vi "Lab01_LabViewSinusoidalWave_Bennett.vi"() -> ()   [LabVIEW 2017]
uses:
  <vilib>/Analysis/baseanly.llb/Mean (DBL).vi
  <vilib>/Analysis/5stat.llb/RMS (DBL).vi
  <vilib>/Analysis/NI_AALBase.lvlib
  <vilib>/Analysis/NI_AALPro.lvlib
panel:
  out "RMS":string
  out "Mean":string
  out "Min":string
  out "Max":string
  in  "Offset":dbl=1.0
  in  "Amplitude":dbl=1.0
  in  "Fraction of Radians":dbl
  in  "milliseconds to wait":u32
  in  "stop":bool
  out "Waveform Graph":dbl[](graph)
  # "09/06/17"
  # "ELEC3800: IoT                               Lab01                                                        Matt Bennett"
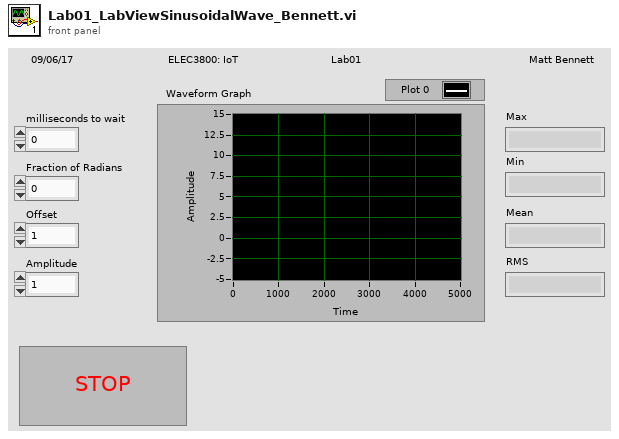
[diagram p1: front panel]
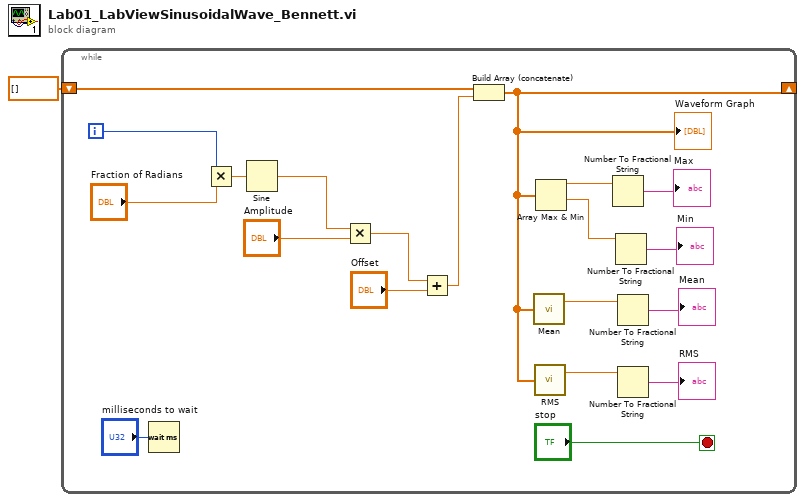
[diagram p0: block diagram]
diagram:
  n1 = while {
    shift-right: [w10] -> _
    shift-left: dbl[] [] -> [w21]
    i -> [w17]
    stop <- "stop" stop-if-true
    n2 = Wait (ms)(milliseconds to wait="milliseconds to wait") -> ()  [unwired: 1 out]
    n3 = Multiply(x=w17, y="Fraction of Radians") -> (x*y=w16:dbl)
    n4 = Sine(x=w16) -> (sin(x)=w14:dbl)
    n5 = Multiply(x=w14, y="Amplitude") -> (x*y=w12:dbl)
    n6 = Add(x=w12, y="Offset") -> (x+y=w11:dbl)
    n7 = Build Array (concatenate)(w21, w11) -> (w10:dbl[])
    "Waveform Graph" <- w10
    n8 = call-poly <vilib>:"Mean.vi"("X"=w10) -> ("mean"=w3:dbl)  [unwired: 1 out]
    n9 = call-poly <vilib>:"RMS.vi"("X"=w10) -> ("rms value"=w2:dbl)  [unwired: 1 out]
    n10 = Array Max & Min(array=w10) -> (max value=w9:dbl, min value=w4:dbl)  [unwired: 2 out]
    n11 = Number To Fractional String(number=w9) -> (F-format string=→"Max":string)  [unwired: 3 in]
    n12 = Number To Fractional String(number=w4) -> (F-format string=→"Min":string)  [unwired: 3 in]
    n13 = Number To Fractional String(number=w3) -> (F-format string=→"Mean":string)  [unwired: 3 in]
    n14 = Number To Fractional String(number=w2) -> (F-format string=→"RMS":string)  [unwired: 3 in]
  }
